vi "lorentzian_fit.vi"(8 "error in (no error)":errorcluster, 11 "power spectrum":cluster{"f0":dbl, "df":dbl, "magnitude":dbl[]}) -> (0 "error out":errorcluster, 3 "Cluster":cluster{"f0":dbl, "df":dbl, "Array":dbl[]})   [LabVIEW 2019]
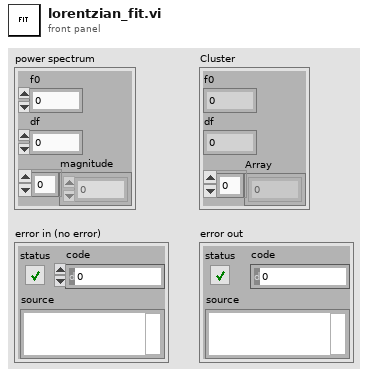
[diagram p1: front panel]
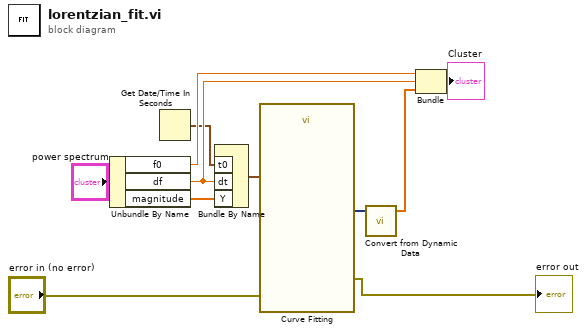
[diagram p0: block diagram]
diagram:
  n1 = Unbundle By Name("power spectrum") -> ("f0"=w8:dbl, "df"=w9:dbl, "magnitude"=w6:dbl[])
  n2 = Get Date/Time In Seconds() -> (seconds since 1Jan1904=w5:timestamp)
  n3 = Bundle By Name("t0"=w5, "dt"=w9, "Y"=w6) -> (w7:waveform(dbl))  [unwired: 1 in]
  n4 = call "Curve Fitting"("error in (no error)"="error in (no error)", "Signals"=w7) -> ("error out"=→"error out":errorcluster, "best fit"=w2:dynamicdata)  [unwired: 5 in, 3 out]
  n5 = call "Convert from Dynamic Data"("Dynamic Data Type"=w2) -> ("Array"=w3:dbl[])  [unwired: 3 in]
  n6 = Bundle("f0"=w8, "df"=w9, "Array"=w3) -> (→"Cluster":cluster{"f0":dbl, "df":dbl, "Array":dbl[]})  [unwired: 1 in]
